vi "Config.vi"(8 "error in (no error)":errorcluster, 11 "AD4212C in":refnum<class "AD4212C.lvclass">) -> (0 "error out":errorcluster, 3 "AD4212C out":refnum<class "AD4212C.lvclass">)   [LabVIEW 2014, in "AD4212C.lvlib" / "AD4212C.lvclass"]
doc: "Abre el VI de Panel de Configuración para que el usuario puede cargar la configuración deseada y permite también Calibrar el dispositivo."
uses:
  AD4212C.lvclass
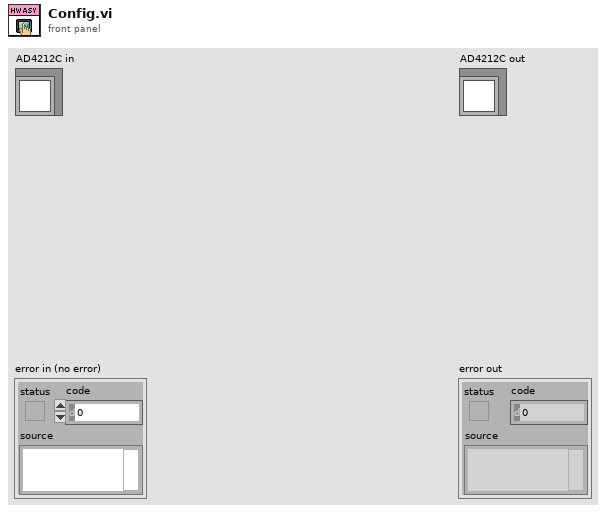
[diagram p1: front panel]
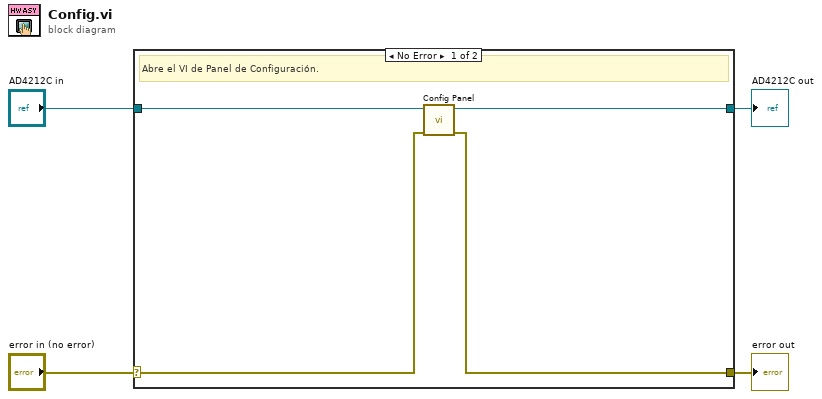
[diagram p0: block diagram]
diagram:
  n1 = case shown="No Error" "error in (no error)" {
    selector: "error in (no error)" -> [w6 w10]
    tunnel: [w5 w10] -> w3
    tunnel: [w7 w9] -> w1
    tunnel: "AD4212C in" -> [w8 w9]
    frame No Error {
      # "Abre el VI de Panel de Configuración."
      n2 = call-dynamic "Config Panel.vi"("error in (no error)"=w6, "AD4212C in"=w8) -> ("error out"=w5:errorcluster, "AD4212C out"=w7:refnum<class "AD4212C.lvclass">)  [unwired: 8 in]
    }
    frame Error {
    }
  }
  "error out" <- w3
  "AD4212C out" <- w1
